vi "Get_Day_File_Summary.vi"(5 "End time":timestamp, 6 "Start time":timestamp, 8 "Data folder location":path) -> ()   [LabVIEW 2020]
uses:
  Anemometry/Anemometry Sub Vis/Globals/Constants_global.vi
  Anemometry/Anemometry Sub Vis/Globals/Preference_global.vi
panel:
  in  "Output Filename":path
  out "Names":string[](array[string])
  out "Summary":string[][](array[string])
  in  "Template":path
  out "Currenly reading":path
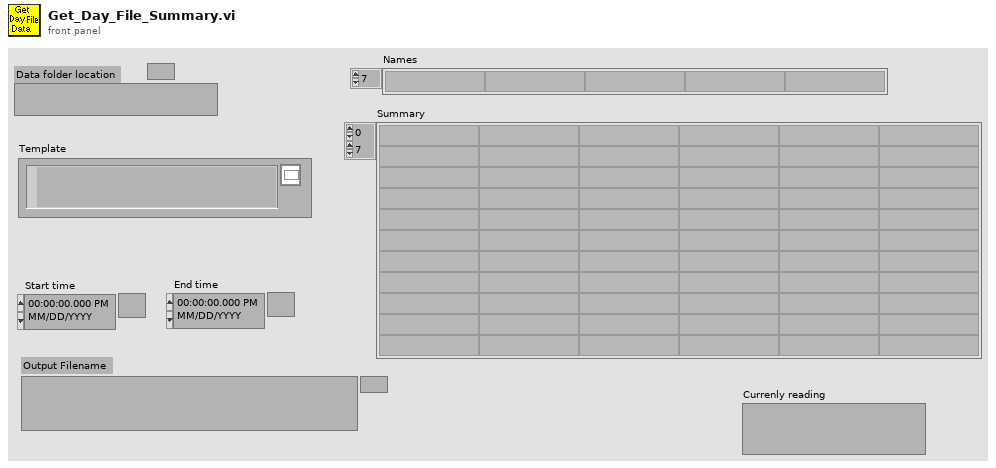
[diagram p1: front panel]
types:
  T1 = enum16{"Show only data summary", "Show data summary", "No data summary"}
  T2 = typedef "LVDateTimeRec.ctl" = cluster{"fractional second":dbl, "second":i32, "minute":i32, "hour":i32, "day of month":i32, "month":i32, "year":i32, "day of week":i32, "day of year":i32, "DST":i32}
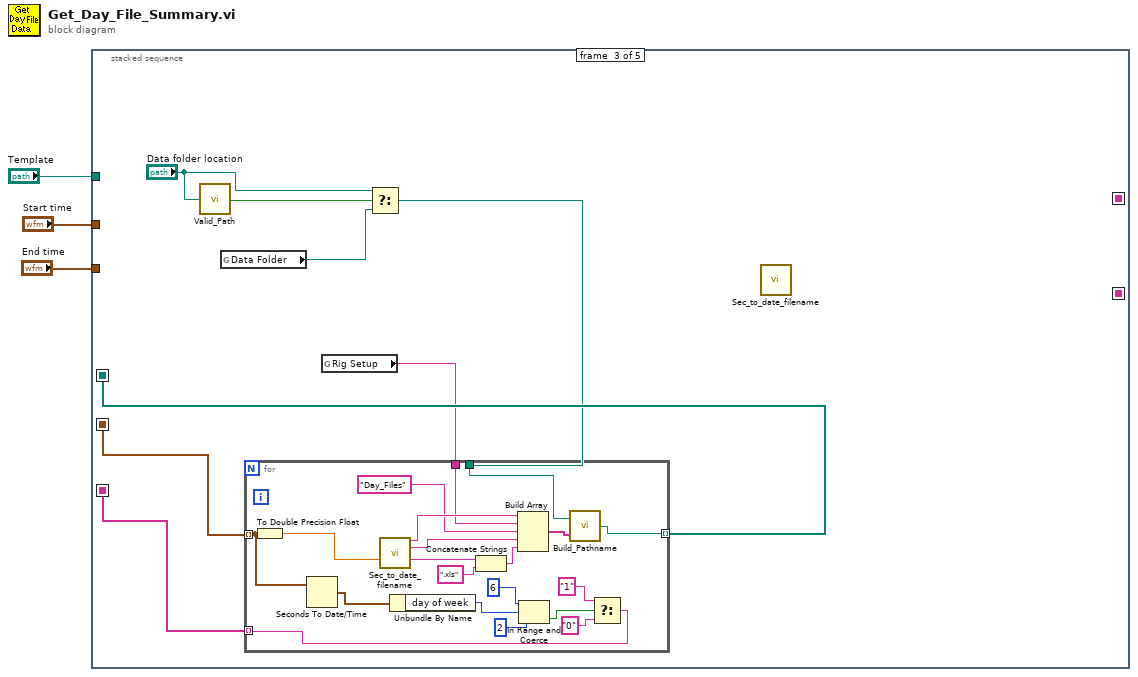
[diagram p0: block diagram]
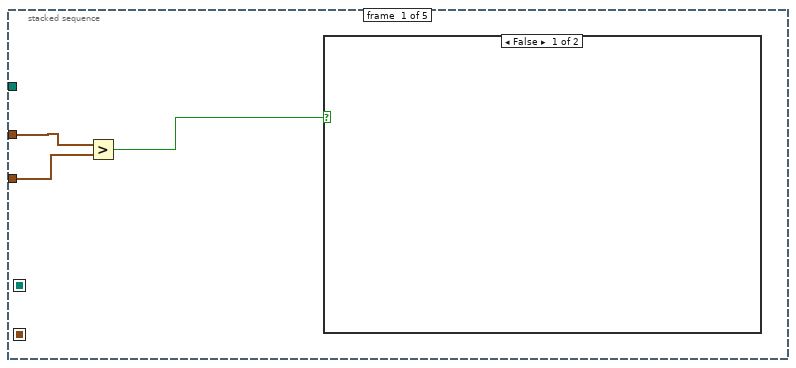
[diagram p2: hidden frame]
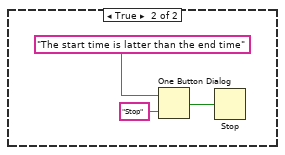
[diagram p3: hidden frame]
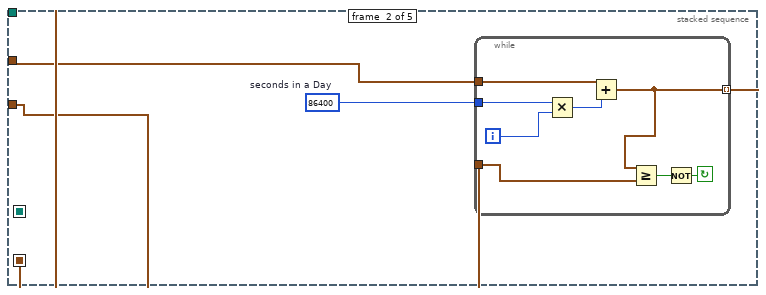
[diagram p4: hidden frame]
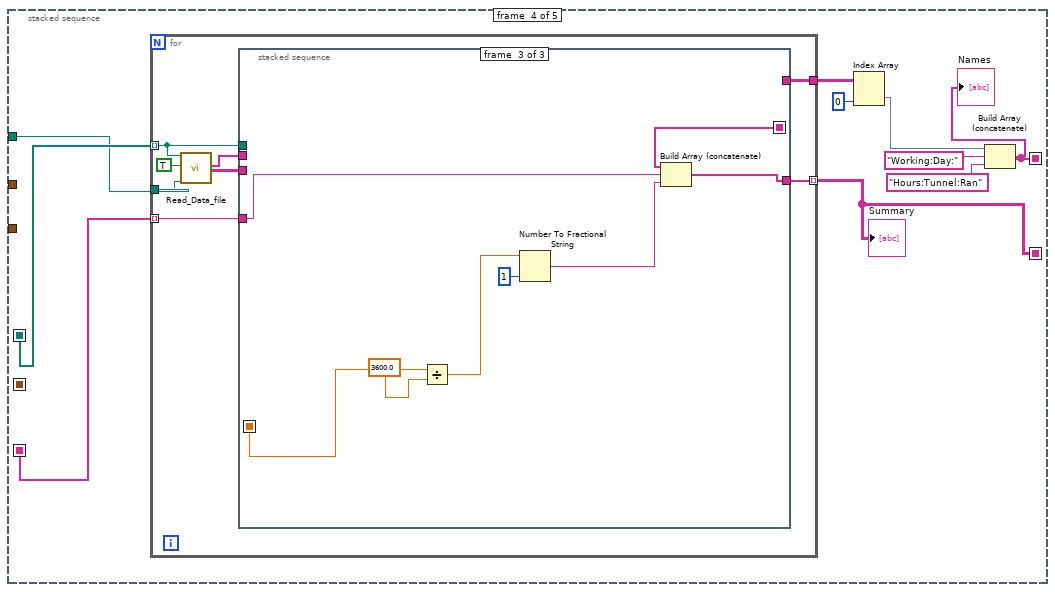
[diagram p5: hidden frame]
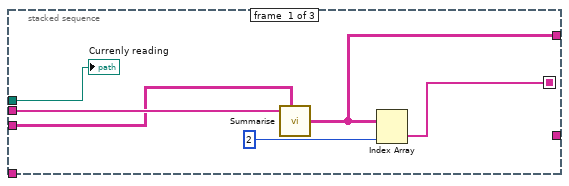
[diagram p6: hidden frame]
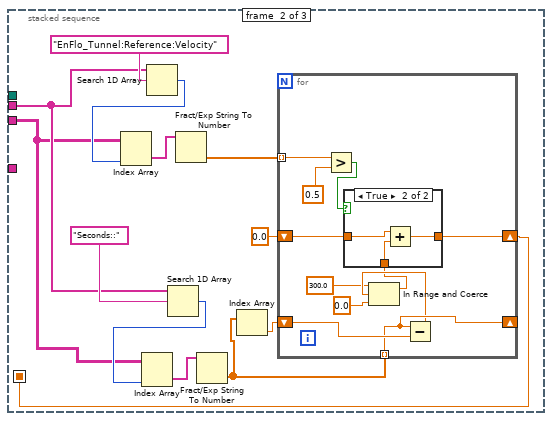
[diagram p7: hidden frame]
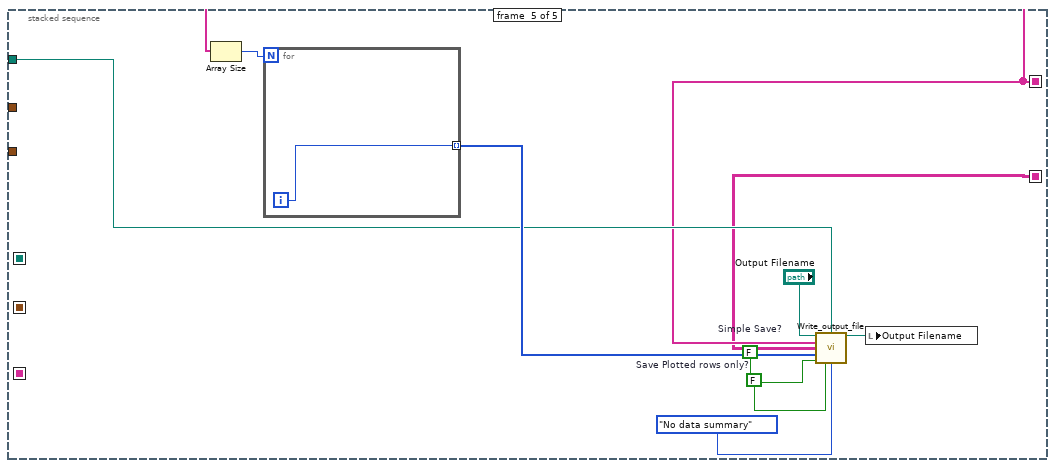
[diagram p9: hidden frame]
diagram:
  n1 = stacked-sequence {
    seq-local: [_ w13 _ _ _] -> [_ _ w29 _ _]
    seq-local: [_ _ w28 _ _] -> [_ _ _ w59 _]
    seq-local: [_ _ w23 _ _] -> [_ _ _ w56 _]
    seq-local: [_ _ _ w50 _] -> [_ _ _ _ w114]
    seq-local: [_ _ _ w51 _] -> [_ _ _ _ w113]
    tunnel: "End time" -> [w5 w10 _ _ _]
    tunnel: "Start time" -> [w4 w11 _ _ _]
    tunnel: "Template" -> [_ _ _ w52 w115]
    frame #0 {
      n2 = Greater?(x=w4, y=w5) -> (0:w6:bool)
      n3 = case shown="False" w6 {
        frame False {
        }
        frame True {
          n4 = One Button Dialog(message="The start time is latter than the end time", button name ("OK")="Stop") -> (true=w8:bool)
          n5 = Stop(stop? (T)=w8) -> ()
        }
      }
    }
    frame #1 {
      w12 = u32 86400  # seconds in a Day
      n6 = while {
        tunnel: [w14] -> w13 mode=indexing
        tunnel: w10 -> [w21]
        tunnel: w11 -> [w15]
        tunnel: w12 -> [w17]
        i -> [w18]
        stop <- w19 continue-if-true
        n7 = Multiply(x=w17, y=w18) -> (x*y=w16:u32)
        n8 = Add(x=w15, y=w16) -> (x+y=w14:timestamp)
        n9 = Greater Or Equal?(x=w14, y=w21) -> (x >= y?=w20:bool)
        n10 = Not(x=w20) -> (.not. x?=w19:bool)
      }
    }
    frame #2 {
      n11 = call "Valid_Path.vi"("Filename"="Data folder location") -> ("Valid Path?"=w27:bool)
      n12 = global read "Constants_global.vi" "Data Folder"() -> (w25:path)
      n13 = global read "Preference_global.vi" "Rig Setup"() -> (w22:string)
      n14 = Select(t="Data folder location", s=w27, f=w25) -> (s? t:f=w24:path)
      n15 = for {
        tunnel: w29 -> [w40] mode=indexing
        tunnel: w24 -> [w45]
        tunnel: [w42] -> w28 mode=indexing
        tunnel: w22 -> [w41]
        tunnel: [w33] -> w23 mode=indexing
        n16 = To Double Precision Float(number=w40) -> (double precision float=w43:dbl)
        n17 = Seconds To Date/Time(time stamp (now)=w40) -> (date time rec=w39:T2)  [unwired: 1 in]
        n18 = call "Sec_to_date_filename.vi"("ss1904"=w43) -> ("YYYY"=w47:string, "mm-YYYY"=w31:string, "DD-mm-YYYY"=w30:string)  [unwired: 5 in, 7 out]
        n19 = Unbundle By Name(w39) -> ("day of week"=w38:i32)
        n20 = Concatenate Strings(w30, ".xls" ("string")) -> (w48:string)
        n21 = Build Array(w47, w41, "Day_Files" ("Input Element"), w31, w48) -> (w44:string[])
        n22 = In Range and Coerce(upper limit=6, x=w38, lower limit=2) -> (In Range?=w35:bool)  [unwired: 1 out]
        n23 = call "Build_Pathname.vi"("PathElements"=w44, "PathnameIn"=w45) -> ("AppendedPath"=w42:path)
        n24 = Select(t="1", s=w35, f="0" ("t")) -> (s? t:f=w33:string)
      }
      n25 = call "Sec_to_date_filename.vi"() -> ()  [unwired: 6 in, 10 out]
    }
    frame #3 {
      n26 = for {
        tunnel: w59 -> [w64] mode=indexing
        tunnel: w52 -> [w63]
        tunnel: [w65] -> w51 mode=indexing
        tunnel: [w67] -> w57
        tunnel: w56 -> [w66] mode=indexing
        n27 = call "Read_Data_file.vi"("Results file"=w64, "Delete First Rows?"=TRUE, "Template File"=w63) -> ("Ch names Out"=w62:string[], "Channel Values Out"=w61:string[][])  [unwired: 4 in, 11 out]
        n28 = stacked-sequence {
          seq-local: [w70 _ _] -> [_ _ w109]
          seq-local: [_ w77 _] -> [_ _ w106]
          tunnel: w64 -> [w73 _ _]
          tunnel: [w71 _ _] -> w67
          tunnel: w66 -> [_ _ w108]
          tunnel: [_ _ w107] -> w65
          tunnel: w62 -> [w69 w80 _]
          tunnel: w61 -> [w68 w79 _]
          frame #0 {
            n29 = call "Summarise.vi"("Channel Names"=w69, "Data"=w68) -> ("Summary"=w71:string[][])  [unwired: 3 in]
            n30 = Index Array(array=w71, index (col)=2 ("disabled index (col)")) -> (element=w70:string[])  [unwired: 1 in]
            "Currenly reading" <- w73
          }
          frame #1 {
            n31 = Search 1D Array(1D array=w80, element="EnFlo_Tunnel:Reference:Velocity") -> (index of element=w85:i32)  [unwired: 1 in]
            n32 = Index Array(array=w79, index (col)=w85) -> (element=w84:string[])  [unwired: 1 in]
            n33 = Search 1D Array(1D array=w80, element="Seconds::") -> (index of element=w82:i32)  [unwired: 1 in]
            n34 = Index Array(array=w79, index (col)=w82) -> (element=w83:string[])  [unwired: 1 in]
            n35 = Fract/Exp String To Number(string=w84) -> (number=w78:dbl[])  [unwired: 3 in, 1 out]
            n36 = Fract/Exp String To Number(string=w83) -> (number=w75:dbl[])  [unwired: 3 in, 1 out]
            n37 = Index Array(array=w75) -> (element=w74:dbl)  [unwired: 1 in]
            n38 = for {
              tunnel: w78 -> [w96] mode=indexing
              shift-right: [w95] -> w77
              shift-left: 0.0 -> [w94]
              tunnel: w75 -> [w91] mode=indexing
              shift-right: [w91] -> _
              shift-left: w74 -> [w92]
              n39 = Greater?(x=w96, y=0.5) -> (0:w93:bool)
              n40 = Subtract(x=w91, y=w92) -> (x-y=w89:dbl)
              n41 = In Range and Coerce(upper limit=300.0, x=w89, lower limit=0.0) -> (coerced(x)=w88:dbl)  [unwired: 1 out]
              n42 = case shown="True" w93 {
                tunnel: [w98 w101] -> w95
                tunnel: w94 -> [w98 w100]
                tunnel: w88 -> [_ w99]
                frame False {
                }
                frame True {
                  n43 = Add(x=w100, y=w99) -> (x+y=w101:dbl)
                }
              }
            }
          }
          frame #2 {
            n44 = Divide(x=w106, y=3600.0) -> (x/y=w104:dbl)
            n45 = Number To Fractional String(number=w104, precision (6)=i16 1) -> (F-format string=w102:string)  [unwired: 2 in]
            n46 = Build Array (concatenate)(w109, w108, w102) -> (w107:string[])
          }
        }
      }
      "Summary" <- w51
      n47 = Index Array(array=w57, index (col)=0 ("disabled index (col)")) -> (element=w55:string[])  [unwired: 1 in]
      n48 = Build Array (concatenate)(w55, "Working:Day:", "Hours:Tunnel:Ran") -> (w50:string[])
      "Names" <- w50
    }
    frame #4 {
      w111 = FALSE  # Save Plotted rows only?
      w112 = FALSE  # Simple Save?
      n49 = Array Size(array=w114) -> (size(s)=w117:i32)
      n50 = for {
        N: w117 -> [_]
        tunnel: [w120] -> w116 mode=indexing
        i -> [w120]
      }
      n51 = call "Write_output_file.vi"("Output filename"="Output Filename", "Template Filename"=w115, "Channel Names"=w114, "Data"=w113, "Desired Columns"=w116, "Simple Save?"=w112, "Save Plotted rows only?"=w111, "Summarise mode"=T1."No data summary") -> ("Output filename Out"=w118:path)  [unwired: 4 in, 3 out]
      n52 = local write "Output Filename"(w118) -> ()
    }
  }
